vi "Load Subpanel.vi"(8 "error in (no error)":errorcluster, 9 "Calling VI":refnum<vi>, 10 "Subpanel Type":T1, 11 "CIF_UI in":refnum<class "CIF_UI.lvclass">) -> (0 "error out":errorcluster, 2 "VI Reference":refnum<vi>, 3 "CIF_UI out":refnum<class "CIF_UI.lvclass">)   [LabVIEW 2021, in "CIF_UI.lvclass"]
uses:
  CIF_UI.lvclass
  Typedef/Subpanel Type.ctl
  CIF_UI.lvclass/CIF_UI.ctl
  Typedef/Subpanel Data.ctl
  CIFCore/Common/Typedef/Errors.ctl
  <vilib>/CIF Foundation/CIF Utilities/Errors/Append Error Location.vi
  <vilib>/Utility/LVLibp/NI_PackedLibraryUtility.lvlib
  CIFUtilities/CIFConfigurationFile/CIF Configuration File.lvlib
  78e05929-4a52-4a7a-a51a-d61806b701c4.vi
  CIFCore/Common/CIFCoreCommon.lvlib
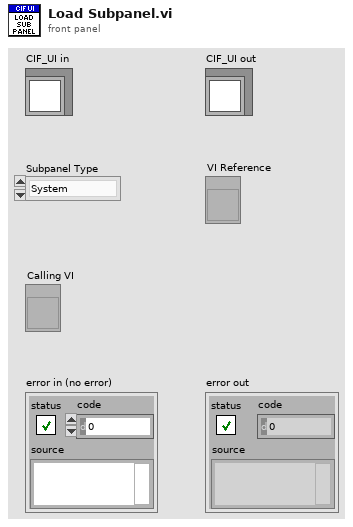
[diagram p1: front panel]
types:
  T1 = typedef "CIF_UI.lvclass/Subpanel Type.ctl" = enum16{"System", "Errors", "Channel", "Plugin"}
  T2 = typedef "CIF_UI.lvclass/Subpanel Data.ctl" = cluster{"VI Reference":refnum<vi>}
  T3 = typedef "CIFCoreCommon.lvlib/Errors.ctl" = enum16{"Invalid Clock ID", "Long Sleep", "gRPC Server Not Found", "Config Parse", "Timestamp Wrap", "Delayed Execution", "Duplicate Channel", "Missing Channel", "Incorrect Type", "Flatten Error", "Unflatten Data", "Unique Name", "Plugin Not Found", "Plugin Type Not Found", "Plugin Version Not Found", "Manager Not Found", "Numerical Issue", "Time Jump", "Clock ID Match", "Channel Length", "Plugin Connection", "gRPC Server Connection", "PPL Name Match", "Build", "Config Log Parse", "Plugin Load", "UI Subpanel Load", "Python Name", "Invalid Name", "Unable to Change Ch Buffer"}
  T4 = typedef "CIF_UI.lvclass/Class Data for SubPanel.ctl" = cluster{"IP Address":string, "Manager gRPC ID":T5, "Server Certificate File (.crt)":path, "Connected":bool, "Manager Connection":bool, "Core UI References":T6, "Subpanel Events":T7}
  T5 = typedef "grpc-lvsupport-release.lvlib/grpcId.ctl" = u64
  T6 = typedef "CIF_UI.lvclass/Core UI References.ctl" = cluster{"Discovered Plugins":refnum<vi>, "Discovered Plugins Valid":bool, "Loaded Plugins":refnum<vi>, "Loaded Plugins Valid":bool, "Publisher Channels":refnum<vi>, "Publisher Channels Valid":bool, "Subscriber Channels":refnum<vi>, "Subscriber Channels Valid":bool, "Plugin Status":refnum<vi>, "Plugin Status Valid":bool, "Channel Connection":refnum<vi>, "Channel Connection Valid":bool, "New Plugin Load":refnum<vi>, "New Plugin Load Valid":bool, "Errors":refnum<vi>, "Errors Valid":bool, "Plugin to Abort":refnum<vi>, "Plugin to Abort Valid":bool, "Connection":refnum<vi>, "Connection Valid":bool, "Exit":refnum<vi>, "Exit Valid":bool, "Run Listen":refnum<vi>, "Run Listen Valid":bool, "CIF Manager Tab":refnum<vi>, "Manger Tab Valid":bool, "Clear Local Error":refnum<vi>, "Clear Local Error Valid":bool, "Local Error":refnum<vi>, "Local Error Valid":bool, "System Errors":refnum<vi>, "System Errors Valid":bool, "Plugin Selection":refnum<vi>, "Plugin Selection Valid":bool}
  T7 = typedef "CIF_UI.lvclass/SubPanel Events.ctl" = cluster{"Clear Local Error":refnum<user-event>, "Shutdown":refnum<user-event>, "gRPC Connection":refnum<user-event>, "Plugin Connection":refnum<user-event>}
  T8 = typedef "CIF_UI.lvclass/Subpanel Map.ctl" = map{T1, T2}
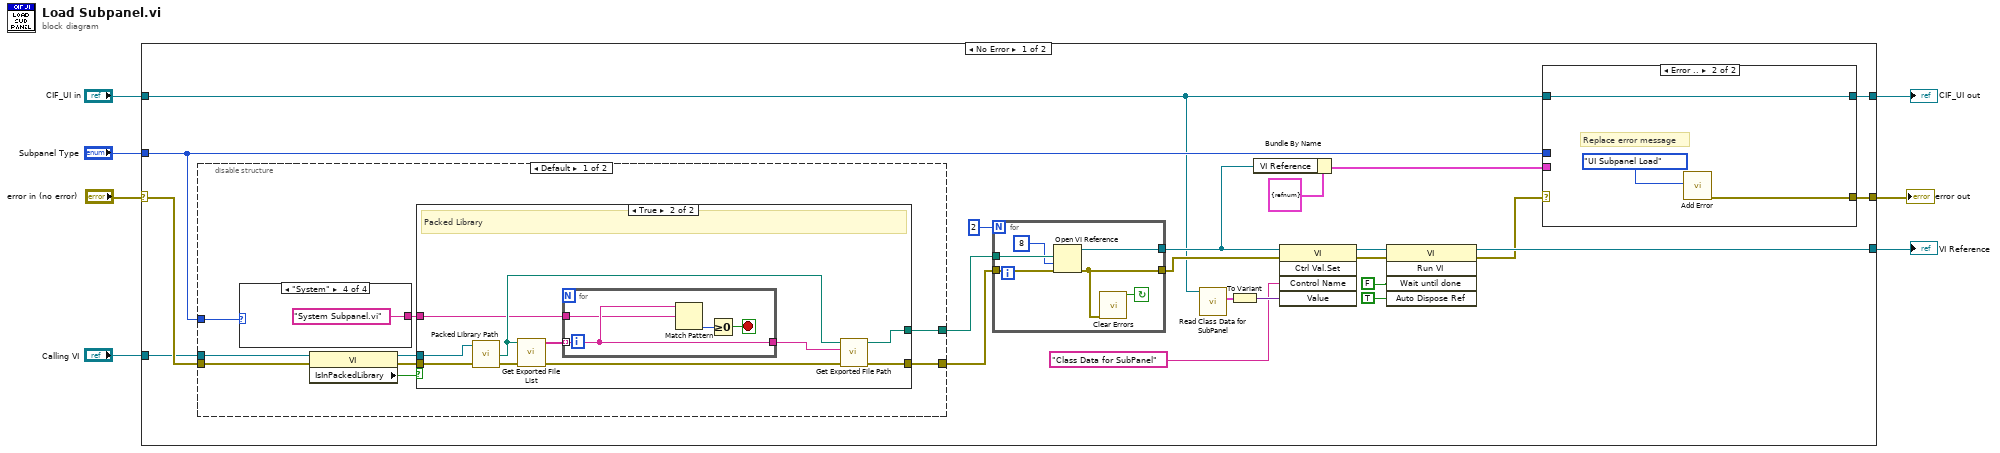
[diagram p0: block diagram]
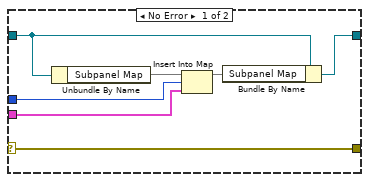
[diagram p2: hidden frame]
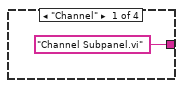
[diagram p3: hidden frame]
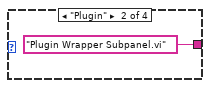
[diagram p4: hidden frame]
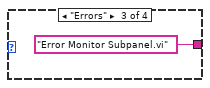
[diagram p5: hidden frame]
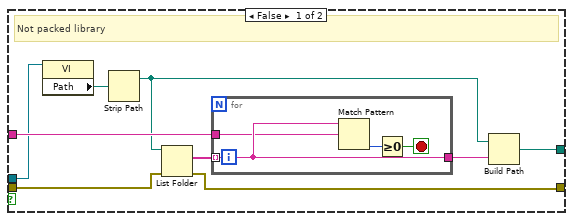
[diagram p6: hidden frame]
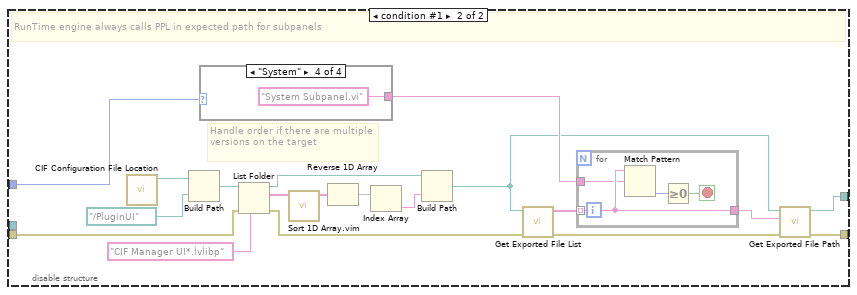
[diagram p7: hidden frame]
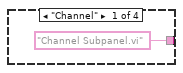
[diagram p8: hidden frame]
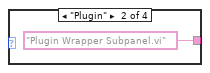
[diagram p9: hidden frame]
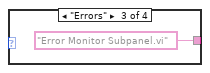
[diagram p10: hidden frame]
diagram:
  n1 = case shown="No Error" "error in (no error)" {
    selector: "error in (no error)" -> [w16 w114]
    tunnel: [w11 w114] -> w6
    tunnel: [w20 w113] -> w4
    tunnel: "CIF_UI in" -> [w9 w113]
    tunnel: "Subpanel Type" -> [w13 _]
    tunnel: [w19 _] -> w2
    tunnel: "Calling VI" -> [w12 _]
    frame No Error {
      n2 = disable-structure shown="Default" {
        disable-tunnel: w16 -> [w45 w81]
        disable-tunnel: [w44 w98] -> w15
        disable-tunnel: [w43 w97] -> w14
        disable-tunnel: w13 -> [w41 w95]
        disable-tunnel: w12 -> [w40 _]
        frame condition #0 (active) {
          n3 = case shown="\"System\"" w41 {
            tunnel: ["Channel Subpanel.vi" ("regular expression") "Plugin Wrapper Subpanel.vi" ("regular expression") "Error Monitor Subpanel.vi" ("regular expression") "System Subpanel.vi" ("regular expression")] -> w42
            frame "Channel" {
            }
            frame "Plugin" {
            }
            frame "Errors" {
            }
            frame "System" {
            }
          }
          n4 = property class="VI"(reference=w40, error in=w45) -> (reference out=w47:refnum<vi>, error out=w48:errorcluster, "IsInPackedLibrary"=w46:bool)
          n5 = case shown="True" w46 {
            tunnel: w47 -> [w55 w75]
            tunnel: w48 -> [w59 w74]
            tunnel: [w53 w66] -> w43
            tunnel: [w58 w68] -> w44
            tunnel: w42 -> [w60 w67]
            frame False {
              # "Not packed library"
              n6 = property class="VI"(reference=w55) -> ("Path"=w56:path)  [unwired: 1 in, 2 out]
              n7 = Strip Path(path=w56) -> (stripped path=w57:path)  [unwired: 1 out]
              n8 = List Folder(path=w57, error in=w59) -> (filenames=w61:string[], error out=w58:errorcluster)  [unwired: 2 in, 2 out]
              n9 = for {
                tunnel: w61 -> [w63] mode=indexing
                tunnel: [w63] -> w54
                tunnel: w60 -> [w62]
                stop <- w64 stop-if-true
                n10 = Match Pattern(string=w63, regular expression=w62) -> (offset past match=w65:i32)  [unwired: 1 in, 3 out]
                n11 = Greater Or Equal To 0?(x=w65) -> (x >= 0?=w64:bool)
              }
              n12 = Build Path(base path=w57, name or relative path=w54) -> (appended path=w53:path)
            }
            frame True {
              # "Packed Library"
              n13 = call <vilib>:"Packed Library Path.vi"("error in (no error)"=w74, "vi reference"=w75) -> ("error out"=w69:errorcluster, "packed library path"=w70:path)  [unwired: 1 in, 1 out]
              n14 = call <vilib>:"Get Exported File List.vi"("error in (no error)"=w69, "packed library path"=w70) -> ("error out"=w72:errorcluster, "qualified names"=w71:string[])  [unwired: 7 in, 1 out]
              n15 = for {
                tunnel: w71 -> [w77] mode=indexing
                tunnel: [w77] -> w73
                tunnel: w67 -> [w76]
                stop <- w78 stop-if-true
                n16 = Match Pattern(string=w77, regular expression=w76) -> (offset past match=w79:i32)  [unwired: 1 in, 3 out]
                n17 = Greater Or Equal To 0?(x=w79) -> (x >= 0?=w78:bool)
              }
              n18 = call <vilib>:"Get Exported File Path.vi"("error in (no error)"=w72, "qualified name"=w73, "packed library path"=w70) -> ("error out"=w68:errorcluster, "path"=w66:path)  [unwired: 7 in]
            }
          }
        }
        frame condition #1 {
          # "Handle order if there are multiple versions on the target"
          # "RunTime engine always calls PPL in expected path for subpanels"
          n19 = call "CIF Configuration File Location.vi"() -> ("configuration file path"=w86:path)  [unwired: 11 in]
          n20 = Build Path(base path=w86, name or relative path=path "../PluginUI") -> (appended path=w85:path)
          n21 = case shown="\"System\"" w95 {
            tunnel: ["Channel Subpanel.vi" ("regular expression") "Plugin Wrapper Subpanel.vi" ("regular expression") "Error Monitor Subpanel.vi" ("regular expression") "System Subpanel.vi" ("regular expression")] -> w96
            frame "Channel" {
            }
            frame "Plugin" {
            }
            frame "Errors" {
            }
            frame "System" {
            }
          }
          n22 = List Folder(path=w85, pattern="CIF Manager UI*.lvlibp", error in=w81) -> (path out=w90:path, filenames=w87:string[], error out=w80:errorcluster)  [unwired: 1 in, 1 out]
          n23 = call "Sort 1D Array.vim"("unsorted array"=w87) -> ("sorted array"=w88:string[])  [unwired: 10 in]
          n24 = Reverse 1D Array(array=w88) -> (reversed array=w89:string[])
          n25 = Index Array(array=w89) -> (element=w91:string)  [unwired: 1 in]
          n26 = Build Path(base path=w90, name or relative path=w91) -> (appended path=w82:path)
          n27 = call <vilib>:"Get Exported File List.vi"("error in (no error)"=w80, "packed library path"=w82) -> ("error out"=w93:errorcluster, "qualified names"=w92:string[])  [unwired: 7 in, 1 out]
          n28 = for {
            tunnel: w92 -> [w100] mode=indexing
            tunnel: [w100] -> w94
            tunnel: w96 -> [w99]
            stop <- w101 stop-if-true
            n29 = Match Pattern(string=w100, regular expression=w99) -> (offset past match=w102:i32)  [unwired: 1 in, 3 out]
            n30 = Greater Or Equal To 0?(x=w102) -> (x >= 0?=w101:bool)
          }
          n31 = call <vilib>:"Get Exported File Path.vi"("error in (no error)"=w93, "qualified name"=w94, "packed library path"=w82) -> ("error out"=w98:errorcluster, "path"=w97:path)  [unwired: 7 in]
        }
      }
      n32 = for {
        N: 2 -> [_]
        tunnel: w14 -> [w112]
        tunnel: [w111] -> w18
        tunnel: [w109] -> w26
        tunnel: w15 -> [w107]
        stop <- w108 continue-if-true
        n33 = Open VI Reference(vi path=w112, options=8, error in (no error)=w107) -> (vi reference=w111:refnum<vi>, error out=w109:errorcluster)  [unwired: 3 in]
        n34 = call <vilib>:"Clear Errors.vi"("error in (no error)"=w109) -> ("specific error cleared?"=w108:bool)  [unwired: 5 in, 1 out]
      }
      n35 = call "Read Class Data for SubPanel.vi"("CIF_UI in"=w9) -> ("Class Data for SubPanel"=w17:T4)  [unwired: 8 in, 2 out]
      n36 = To Variant(anything=w17) -> (Variant=w22:variant)
      n37 = Bundle By Name(cluster=T2 {"VI Reference"=refnum} ("SubPanel Data"), "VI Reference"=w18) -> (w21:T2)
      n38 = invoke class="VI" method="Ctrl Val.Set"(reference=w18, error in=w26, "Control Name"="Class Data for SubPanel", "Value"=w22) -> (reference out=w27:refnum<vi>, error out=w28:errorcluster)  [unwired: 1 in, 3 out]
      n39 = invoke class="VI" method="Run VI"(reference=w27, error in=w28, "Wait until done"=FALSE ("Wait Until Done"), "Auto Dispose Ref"=TRUE ("Auto Dispose Reference")) -> (reference out=w19:refnum<vi>, error out=w8:errorcluster)  [unwired: 1 in, 3 out]
      n40 = case shown="Error .." w8 {
        selector: w8 -> [w30 _]
        tunnel: w21 -> [w35 _]
        tunnel: [w33 w39] -> w20
        tunnel: w13 -> [w32 _]
        tunnel: [w30 w38] -> w11
        tunnel: w9 -> [w31 w39]
        frame No Error {
          n41 = Unbundle By Name(w31) -> ("Subpanel Map"=w36:T8)
          n42 = Insert Into Map(map in=w36, key=w32, value=w35) -> (map out=w34:T8)  [unwired: 2 out]
          n43 = Bundle By Name(cluster=w31, "Subpanel Map"=w34) -> (w33:refnum<class "CIF_UI.lvclass">)
        }
        frame Error {
          # "Replace error message"
          n44 = call "Add Error.vi"("Error"=Errors."UI Subpanel Load") -> ("error out"=w38:errorcluster)  [unwired: 10 in]
        }
      }
    }
    frame Error {
    }
  }
  "error out" <- w6
  "CIF_UI out" <- w4
  "VI Reference" <- w2
